vi "Host to Minion ID.vi"(10 "hostname":string) -> (2 "minion ID":string)   [LabVIEW 2018]
uses:
  <vilib>/httpClient/POSTBuffer.vi
  <vilib>/httpClient/LabVIEWHTTPClient.lvlib
panel:
  in  "server":string
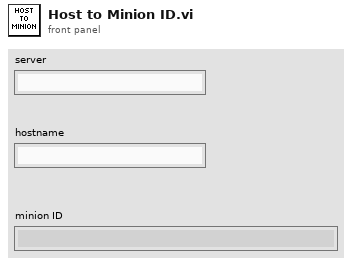
[diagram p1: front panel]
types:
  T1 = cluster{"status_code":i32, "result":cluster{"_id":cluster{"$oid":string}, "id":string}[]}
  T2 = typedef "LabVIEWHTTPClient.lvlib/ClientHandle.ctl" = refnum<k1>
  T3 = cluster{"_id":cluster{"$oid":string}, "id":string}[]
  T4 = cluster{"_id":cluster{"$oid":string}, "id":string}
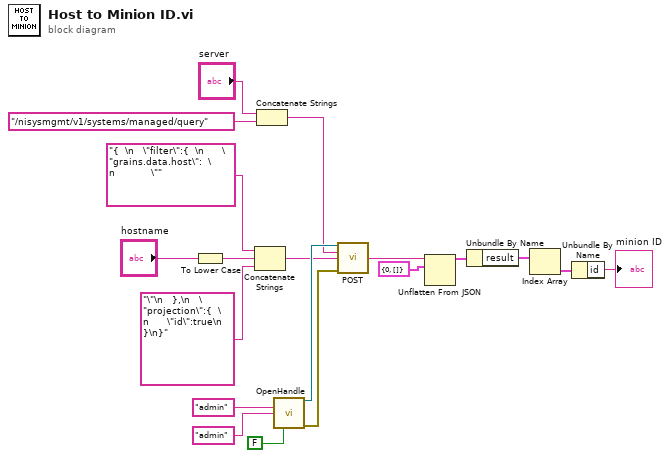
[diagram p0: block diagram]
diagram:
  n1 = To Lower Case(string="hostname") -> (all lower case string=w7:string)
  n2 = Concatenate Strings("{  \n   \"filter\":{  \n      \"grains.data.host\":  \n            \"", w7, "\"\n   },\n   \"projection\":{  \n      \"id\":true\n   }\n}" ("string")) -> (w10:string)
  n3 = Concatenate Strings("server", "/nisysmgmt/v1/systems/managed/query" ("string")) -> (w14:string)
  n4 = call <vilib>:"OpenHandle.vi"("username"="admin", "password"="admin", "verify server(true)"=FALSE) -> ("client handle out"=w19:T2, "error out"=w18:errorcluster)  [unwired: 11 in]
  n5 = call-poly <vilib>:"POST.vi"("client handle"=w19, "url"=w14, "buffer"=w10, "error in (no error)"=w18) -> ("body"=w6:string)  [unwired: 8 in, 3 out]
  n6 = Unflatten From JSON(JSON string=w6, type and defaults=T1 {"status_code"=0, "result"=[]}) -> (value=w4:T1)  [unwired: 5 in, 1 out]
  n7 = Unbundle By Name(w4) -> ("result"=w3:T3)
  n8 = Index Array(array=w3) -> (element=w2:T4)  [unwired: 1 in]
  n9 = Unbundle By Name(w2) -> ("id"=→"minion ID":string)
